vi "五参数标样核查.vi"(11 "启动参数":T1={"测量模式"=enum."水样测试", "数据标记表"="N", "输出参数"={"水温"=FALSE, "pH"=FALSE, "DO"=FALSE, "浊度"=FALSE, "电导率"=FALSE, "保存组数"=0.0}}) -> ()   [LabVIEW 2016, in "斯坦道多参数.lvlib"]
panel:
  out "枚举":T2(ring)
  out "状态":string
  out "数值":i32
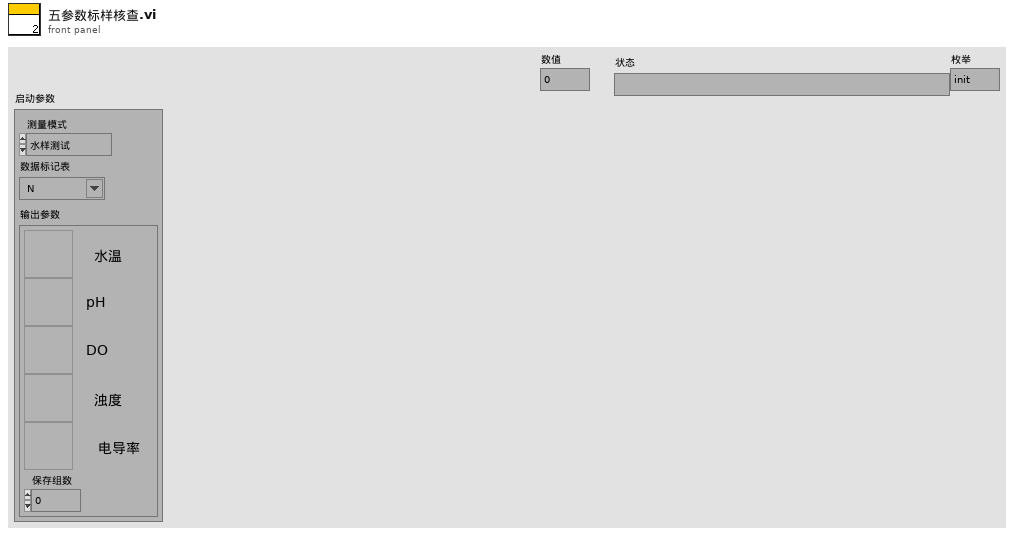
[diagram p1: front panel]
types:
  T1 = cluster{"测量模式":enum16{"待机", "水样测试", "标样核查", "零点核查", "跨度核查", "空白测试", "平行样测试", "加标回收", "空白校准", "标样校准", "初始化（清洗）"}, "数据标记表":string, "输出参数":cluster{"水温":bool, "pH":bool, "DO":bool, "浊度":bool, "电导率":bool, "保存组数":dbl}}
  T2 = enum16{"init", "开机", "启动测量", "读取测量值", "存储数据", "关闭测量", "关机", "结束"}
  T3 = cluster{"时间标识":timestamp, "设备":string, "日志信息":string, "流程参数":string}
  T4 = cluster{"系统时间":timestamp, "工作状态":u16, "测量模式":u16, "告警代码":enum16{"无告警", "缺试剂告警", "缺水样告警", "缺蒸馏水告警", "缺标液告警", "仪表漏液告警", "标定异常告警", "超量程告警", "加热异常", "低试剂预警", "超上限告警", "超下限告警", "仪表内部其他异常", "滴定异常告警", "电极异常告警", "量程切换告警", "参数设置告警", "PH电极电位异常", "电导率电极异常", "浊度光度异常", "溶解氧电极异常", "溶解氧光强异常", "温度异常告警", "PH异常告警", "溶解氧异常告警", "电导率异常告警", "浊度异常告警", "叶绿素异常告警", "藻密度异常告警", "蓝绿藻异常告警", "ORP异常告警", "氨氮异常告警", "清洁刷异常告警", "SD卡异常告警", "蓝牙异常告警", "Wifi异常告警", "流程异常告警"}, "故障代码":enum16{"无故障", "电机故障", "温度故障", "通讯故障", "滴定故障"}, "日志代码":u16, "软件版本":string}
  T5 = enum16{"待机", "水样测试", "标样核查", "零点核查", "跨度核查", "空白测试", "平行样测试", "加标回收", "空白校准", "标样校准", "初始化（清洗）"}
  T6 = cluster{"数据标记表":string, "测量模式":enum16{"待机", "水样测试", "标样核查", "零点核查", "跨度核查", "空白测试", "平行样测试", "加标回收", "空白校准", "标样校准", "初始化（清洗）"}, "database":string}
  T7 = cluster{"水温标准液标准浓度":dbl, "酸碱度标准液标准浓度":dbl, "溶解氧标准液标准浓度":dbl, "电导率标准液标准浓度":dbl, "浊度标准液标准浓度":dbl}
  T8 = cluster{"因子编码":string, "单位":string, "标样参考值":sgl, "水样数据时间":timestamp, "水样实测值":sgl, "水样数据标识":string, "K":sgl, "B":sgl, "T":sgl, "H":sgl, "水深":sgl, "探头温度":sgl}
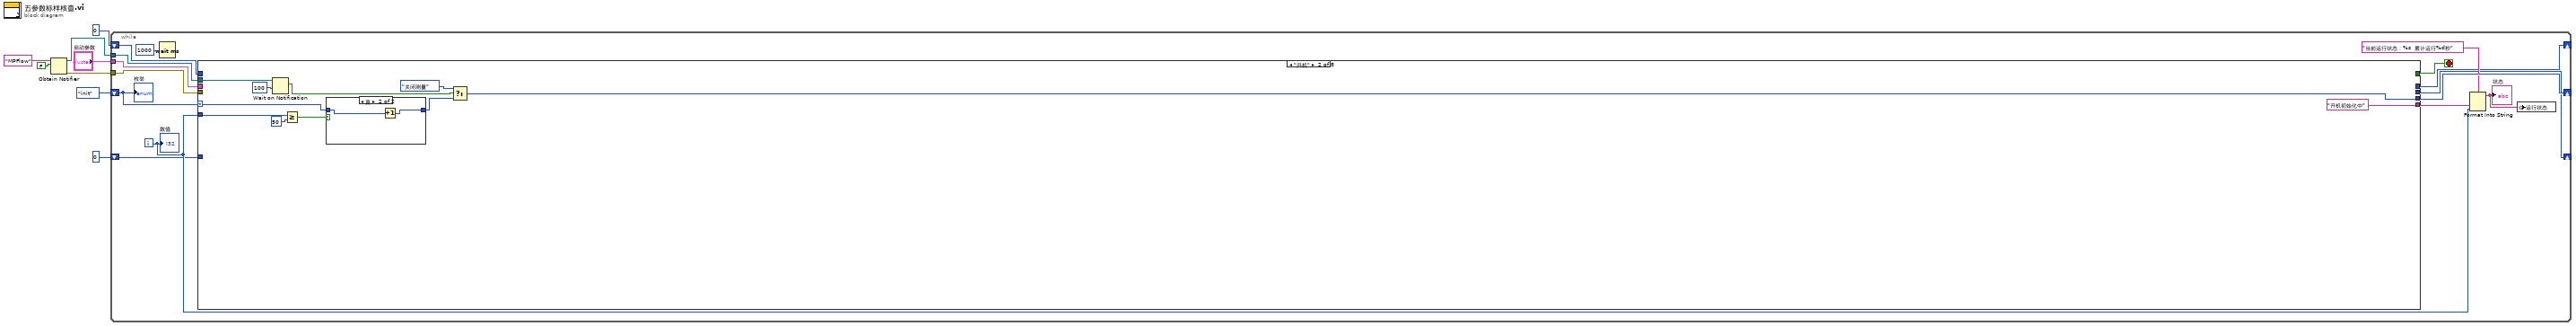
[diagram p0: block diagram]
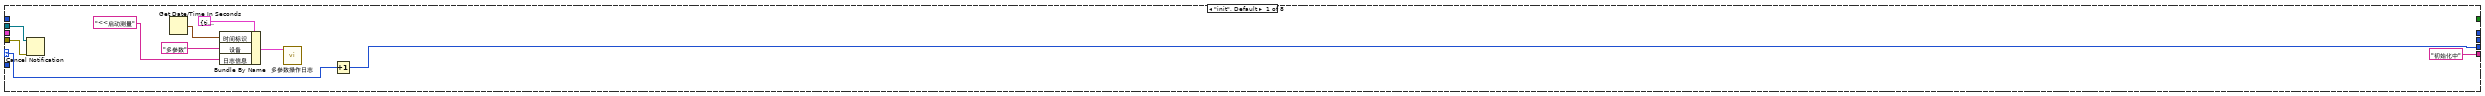
[diagram p2: hidden frame]
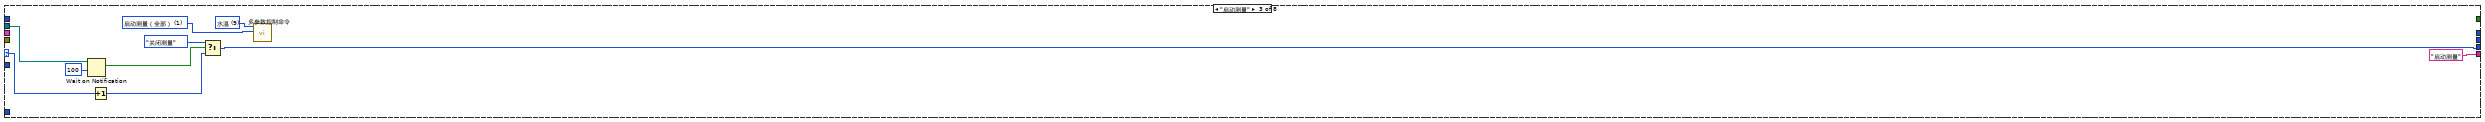
[diagram p4: hidden frame]
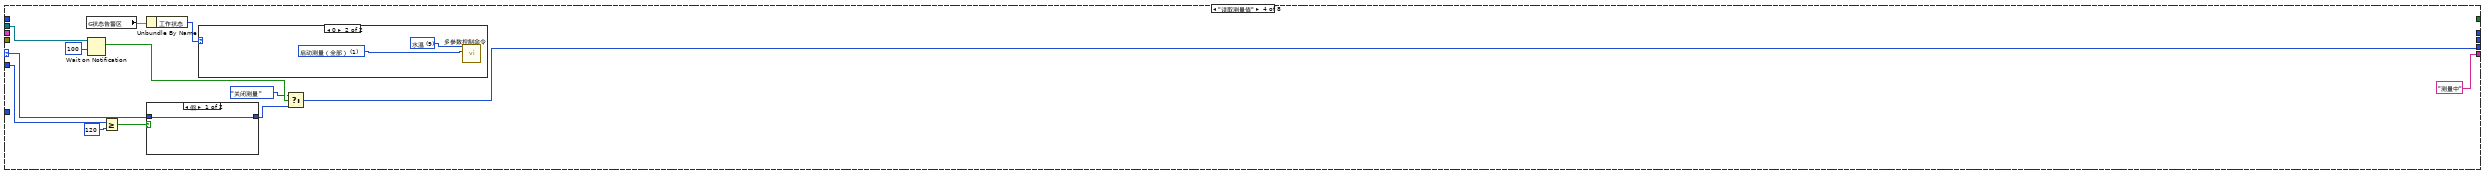
[diagram p5: hidden frame]
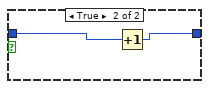
[diagram p7: hidden frame]
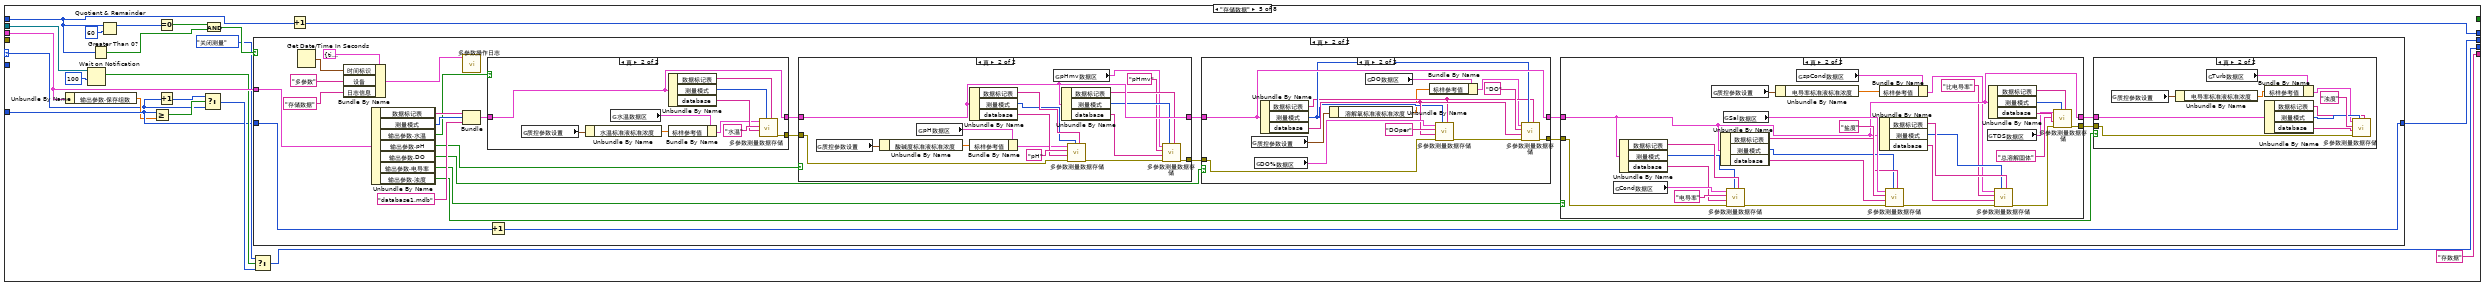
[diagram p8: hidden frame]
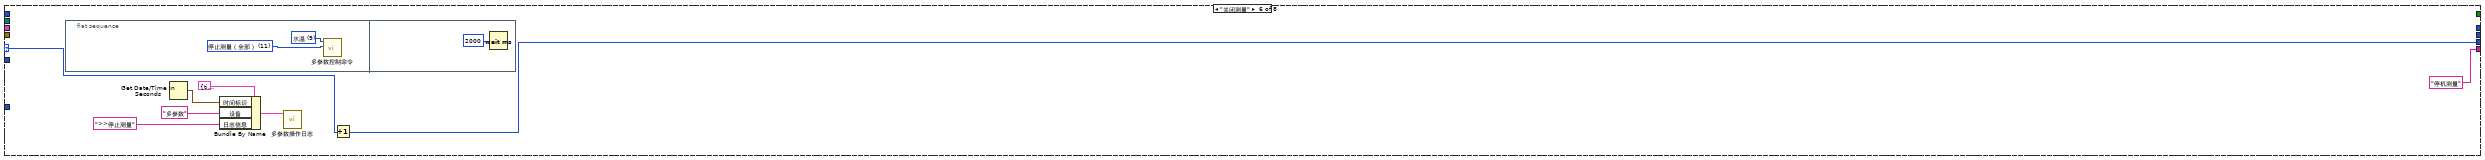
[diagram p15: hidden frame]
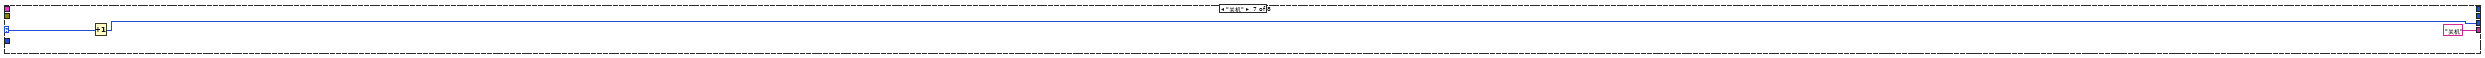
[diagram p16: hidden frame]
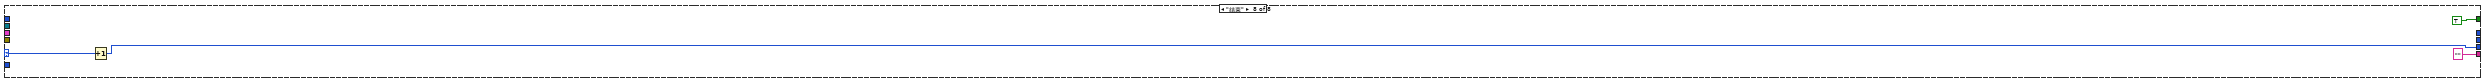
[diagram p17: hidden frame]
diagram:
  n1 = Obtain Notifier(name (unnamed)="MPFlow" ("名称（未命名）"), notification data type=FALSE) -> (notifier out=w5:refnum<notifier>, error out=w4:errorcluster)  [unwired: 2 in, 1 out]
  n2 = while {
    shift-right: [w19] -> _
    shift-left: T2."init" ("枚举") -> [w23]
    tunnel: w5 -> [w21]
    tunnel: w4 -> [w20]
    tunnel: "启动参数" -> [w13]
    shift-right: [w11] -> _
    shift-left: u32 0 ("等待时间（毫秒）") -> [w12]
    shift-right: [w9] -> _
    shift-left: u32 0 ("等待时间（毫秒）") -> [w10]
    i -> [w15]
    stop <- w22 stop-if-true
    n3 = Wait (ms)(milliseconds to wait=u32 1000 ("等待时间（毫秒）")) -> ()  [unwired: 1 out]
    n4 = case shown="\"开机\"" w23 {
      selector: w23 -> [w31 w44 w57 w70 w76 w214 w220 w223]
      tunnel: [_ _ _ _ _ _ _ TRUE] -> w22
      tunnel: w21 -> [w33 w39 w56 w67 w86 _ _ _]
      tunnel: w20 -> [w32 _ _ _ _ _ _ _]
      tunnel: [w30 w37 w53 w65 w82 w213 w219 w222] -> w19
      tunnel: w15 -> [_ w43 _ w60 _ _ _ _]
      tunnel: ["初始化中" ("状态") "开机初始化中" ("状态") "启动测量" ("状态") "测量中" ("状态") "存数据" ("状态") "停机测量" ("状态") "关机" ("状态") "" ("状态")] -> w16
      tunnel: w13 -> [_ _ _ _ w95 _ _ _]
      tunnel: w12 -> [_ _ _ _ w89 _ _ _]
      tunnel: [_ _ _ _ w90 _ _ _] -> w11
      tunnel: w10 -> [_ _ _ _ w79 _ _ _]
      tunnel: [_ _ _ _ w81 _ _ _] -> w9
      frame "init", Default {
        n5 = Cancel Notification(0:w33, 3:w32) -> ()  [unwired: 3 out]
        n6 = Get Date/Time In Seconds() -> (seconds since 1Jan1904=w27:timestamp)
        n7 = Bundle By Name(cluster=T3 {"时间标识"=timestamp(0 s since 1904-01-01), "设备"="", "日志信息"="", "流程参数"=""} ("data in"), "时间标识"=w27, "设备"="多参数", "日志信息"="<<启动测量") -> (w26:T3)
        n8 = call "多参数操作日志.vi"("data in"=w26) -> ()  [unwired: 10 in, 1 out]
        n9 = Increment(x=w31) -> (x+1=w30:T2)
      }
      frame "开机" {
        n10 = Wait on Notification(notifier=w39, timeout in ms (-1)=100 ("超时毫秒(-1)")) -> (notification=w40:bool)  [unwired: 2 in, 3 out]
        n11 = Greater Or Equal?(x=w43, y=50) -> (x >= y?=w41:bool)
        n12 = case shown="真" w41 {
          tunnel: w44 -> [w45 w47]
          tunnel: [w45 w46] -> w38
          frame False {
          }
          frame True {
            n13 = Increment(x=w47) -> (x+1=w46:T2)
          }
        }
        n14 = Select(t=T2."关闭测量" ("枚举"), s=w40, f=w38) -> (s? t:f=w37:T2)
      }
      frame "启动测量" {
        w48 = u16 1 items=["启动测量（全部）"=1, "初始化（清洗）"=10, "停止测量（全部）"=11, "校时"=13, "启动测量（单个传感器）"=19, "停止测量（单个传感器）"=20] ("控制命令")
        w49 = u16 9 items=["氨氮"=3, "水温"=9, "pH值"=10, "溶解氧"=11, "电导率"=12, "浊度"=13, "叶绿素a"=14, "藻密度"=15, "蓝绿藻"=16, "氧化还原电位"=17, "溶解氧%"=18, "盐度"=19] ("站号")
        n15 = Wait on Notification(notifier=w56, timeout in ms (-1)=100 ("超时毫秒(-1)")) -> (notification=w55:bool)  [unwired: 2 in, 3 out]
        n16 = Increment(x=w57) -> (x+1=w54:T2)
        n17 = Select(t=T2."关闭测量" ("枚举"), s=w55, f=w54) -> (s? t:f=w53:T2)
        n18 = call "多参数控制命令.vi"("控制命令"=w48, "站号"=w49) -> ()  [unwired: 9 in, 1 out]
      }
      frame "读取测量值" {
        n19 = global read "多参数全局变量.vi" "状态告警区"() -> (w59:T4)
        n20 = Wait on Notification(notifier=w67, timeout in ms (-1)=100 ("超时毫秒(-1)")) -> (notification=w68:bool)  [unwired: 2 in, 3 out]
        n21 = Greater Or Equal?(x=w60, y=120) -> (x >= y?=w69:bool)
        n22 = Unbundle By Name(w59) -> ("工作状态"=w58:u16)
        n23 = case shown="假" w69 {
          tunnel: w70 -> [w73 w75]
          tunnel: [w73 w74] -> w66
          frame False {
          }
          frame True {
            n24 = Increment(x=w75) -> (x+1=w74:T2)
          }
        }
        n25 = case shown="0" w58 {
          frame Default {
          }
          frame 0 {
            w71 = u16 1 items=["启动测量（全部）"=1, "初始化（清洗）"=10, "停止测量（全部）"=11, "校时"=13, "启动测量（单个传感器）"=19, "停止测量（单个传感器）"=20] ("控制命令")
            w72 = u16 9 items=["氨氮"=3, "水温"=9, "pH值"=10, "溶解氧"=11, "电导率"=12, "浊度"=13, "叶绿素a"=14, "藻密度"=15, "蓝绿藻"=16, "氧化还原电位"=17, "溶解氧%"=18, "盐度"=19] ("站号")
            n26 = call "多参数控制命令.vi"("控制命令"=w71, "站号"=w72) -> ()  [unwired: 9 in, 1 out]
          }
        }
        n27 = Select(t=T2."关闭测量" ("枚举"), s=w68, f=w66) -> (s? t:f=w65:T2)
      }
      frame "存储数据" {
        n28 = Unbundle By Name(w95) -> ("输出参数.保存组数"=w78:dbl)
        n29 = Wait on Notification(notifier=w86, timeout in ms (-1)=100 ("超时毫秒(-1)")) -> (notification=w85:bool)  [unwired: 2 in, 3 out]
        n30 = Greater Than 0?(x=w89) -> (x > 0?=w88:bool)
        n31 = Quotient & Remainder(x=w89, y=u32 60) -> (x-y*floor(x/y)=w93:u32)  [unwired: 1 out]
        n32 = Greater Or Equal?(x=w79, y=w78) -> (x >= y?=w80:bool)
        n33 = Equal To 0?(x=w93) -> (x = 0?=w92:bool)
        n34 = Increment(x=w76) -> (x+1=w77:T2)
        n35 = Select(t=w77, s=w80, f=w76) -> (s? t:f=w84:T2)
        n36 = Compound Arithmetic op=AND ("复合运算")(w92, w88) -> (w91:bool)
        n37 = case shown="真" w91 {
          tunnel: w95 -> [_ w122]
          tunnel: w79 -> [w97 w99]
          tunnel: [w97 w98] -> w81
          frame False {
          }
          frame True {
            n38 = Get Date/Time In Seconds() -> (seconds since 1Jan1904=w108:timestamp)
            n39 = Bundle By Name(cluster=T3 {"时间标识"=timestamp(0 s since 1904-01-01), "设备"="", "日志信息"="", "流程参数"=""} ("data in"), "时间标识"=w108, "设备"="多参数", "日志信息"="存储数据") -> (w107:T3)
            n40 = Unbundle By Name(w122) -> ("数据标记表"=w116:string, "测量模式"=w115:T5, "输出参数.水温"=w104:bool, "输出参数.pH"=w103:bool, "输出参数.DO"=w102:bool, "输出参数.电导率"=w101:bool, "输出参数.浊度"=w100:bool)
            n41 = call "多参数操作日志.vi"("data in"=w107) -> ()  [unwired: 10 in, 1 out]
            n42 = Bundle("数据标记表"=w116, "测量模式"=w115, "database"="database1.mdb") -> (w114:T6)  [unwired: 1 in]
            n43 = case shown="真" w104 {
              tunnel: [_ w205] -> w121
              tunnel: w114 -> [w196 w204]
              tunnel: [w196 w204] -> w113
              frame False {
              }
              frame True {
                n44 = global read "多参数断电保存全局变量.vi" "质控参数设置"() -> (w199:T7)
                n45 = Unbundle By Name(w199) -> ("水温标准液标准浓度"=w198:dbl)
                n46 = global read "多参数全局变量.vi" "水温数据区"() -> (w200:T8)
                n47 = Unbundle By Name(w204) -> ("数据标记表"=w203:string, "测量模式"=w202:T5, "database"=w201:string)
                n48 = Bundle By Name(cluster=w200, "标样参考值"=w198) -> (w197:T8)
                n49 = call "多参数测量数据存储.vi"("数据标记表"=w203, "测量模式"=w202, "database"=w201, "table输入"="水温", "data in"=w197) -> ("error out"=w205:errorcluster)  [unwired: 6 in]
              }
            }
            n50 = Increment(x=w99) -> (x+1=w98:u32)
            n51 = case shown="真" w103 {
              tunnel: w121 -> [_ w195]
              tunnel: [_ w185] -> w120
              tunnel: w113 -> [w178 w190]
              tunnel: [w178 w190] -> w111
              frame False {
              }
              frame True {
                n52 = global read "多参数断电保存全局变量.vi" "质控参数设置"() -> (w182:T7)
                n53 = Unbundle By Name(w182) -> ("酸碱度标准液标准浓度"=w181:dbl)
                n54 = global read "多参数全局变量.vi" "pH数据区"() -> (w180:T8)
                n55 = Unbundle By Name(w190) -> ("数据标记表"=w193:string, "测量模式"=w192:T5, "database"=w191:string)
                n56 = Bundle By Name(cluster=w180, "标样参考值"=w181) -> (w179:T8)
                n57 = global read "多参数全局变量.vi" "pHmv数据区"() -> (w184:T8)
                n58 = Unbundle By Name(w190) -> ("数据标记表"=w189:string, "测量模式"=w188:T5, "database"=w187:string)
                n59 = call "多参数测量数据存储.vi"("数据标记表"=w193, "测量模式"=w192, "error in (no error)"=w195, "database"=w191, "table输入"="pH", "data in"=w179) -> ("error out"=w186:errorcluster)  [unwired: 5 in]
                n60 = call "多参数测量数据存储.vi"("数据标记表"=w189, "测量模式"=w188, "error in (no error)"=w186, "database"=w187, "table输入"="pHmv", "data in"=w184) -> ("error out"=w185:errorcluster)  [unwired: 5 in]
              }
            }
            n61 = case shown="真" w102 {
              tunnel: w120 -> [_ w177]
              tunnel: [_ w174] -> w119
              tunnel: [w163 w171] -> w112
              tunnel: w111 -> [w163 w171]
              frame False {
              }
              frame True {
                n62 = global read "多参数断电保存全局变量.vi" "质控参数设置"() -> (w167:T7)
                n63 = global read "多参数全局变量.vi" "DO%数据区"() -> (w173:T8)
                n64 = Unbundle By Name(w171) -> ("数据标记表"=w168:string, "测量模式"=w169:T5, "database"=w170:string)
                n65 = Unbundle By Name(w167) -> ("溶解氧标准液标准浓度"=w166:dbl)
                n66 = global read "多参数全局变量.vi" "DO数据区"() -> (w165:T8)
                n67 = Bundle By Name(cluster=w165, "标样参考值"=w166) -> (w164:T8)
                n68 = call "多参数测量数据存储.vi"("数据标记表"=w168, "测量模式"=w169, "error in (no error)"=w177, "database"=w170, "table输入"="DOper", "data in"=w173) -> ("error out"=w176:errorcluster)  [unwired: 5 in]
                n69 = call "多参数测量数据存储.vi"("数据标记表"=w168, "测量模式"=w169, "error in (no error)"=w176, "database"=w170, "table输入"="DO", "data in"=w164) -> ("error out"=w174:errorcluster)  [unwired: 5 in]
              }
            }
            n70 = case shown="真" w101 {
              tunnel: w119 -> [_ w160]
              tunnel: [_ w141] -> w118
              tunnel: w112 -> [w133 w150]
              tunnel: [w133 w150] -> w110
              frame False {
              }
              frame True {
                n71 = global read "多参数全局变量.vi" "Cond数据区"() -> (w162:T8)
                n72 = Unbundle By Name(w150) -> ("数据标记表"=w155:string, "测量模式"=w154:T5, "database"=w156:string)
                n73 = global read "多参数断电保存全局变量.vi" "质控参数设置"() -> (w137:T7)
                n74 = Unbundle By Name(w150) -> ("数据标记表"=w153:string, "测量模式"=w152:T5, "database"=w151:string)
                n75 = global read "多参数全局变量.vi" "Sal数据区"() -> (w158:T8)
                n76 = call "多参数测量数据存储.vi"("数据标记表"=w155, "测量模式"=w154, "error in (no error)"=w160, "database"=w156, "table输入"="电导率", "data in"=w162) -> ("error out"=w159:errorcluster)  [unwired: 5 in]
                n77 = Unbundle By Name(w137) -> ("电导率标准液标准浓度"=w136:dbl)
                n78 = global read "多参数全局变量.vi" "spCond数据区"() -> (w135:T8)
                n79 = Bundle By Name(cluster=w135, "标样参考值"=w136) -> (w134:T8)
                n80 = Unbundle By Name(w150) -> ("数据标记表"=w149:string, "测量模式"=w148:T5, "database"=w147:string)
                n81 = call "多参数测量数据存储.vi"("数据标记表"=w153, "测量模式"=w152, "error in (no error)"=w159, "database"=w151, "table输入"="盐度", "data in"=w158) -> ("error out"=w146:errorcluster)  [unwired: 5 in]
                n82 = global read "多参数全局变量.vi" "TDS数据区"() -> (w140:T8)
                n83 = Unbundle By Name(w150) -> ("数据标记表"=w142:string, "测量模式"=w143:T5, "database"=w144:string)
                n84 = call "多参数测量数据存储.vi"("数据标记表"=w149, "测量模式"=w148, "error in (no error)"=w146, "database"=w147, "table输入"="比电导率", "data in"=w134) -> ("error out"=w145:errorcluster)  [unwired: 5 in]
                n85 = call "多参数测量数据存储.vi"("数据标记表"=w142, "测量模式"=w143, "error in (no error)"=w145, "database"=w144, "table输入"="总溶解固体", "data in"=w140) -> ("error out"=w141:errorcluster)  [unwired: 5 in]
              }
            }
            n86 = case shown="真" w100 {
              tunnel: w118 -> [_ w132]
              tunnel: w110 -> [_ w130]
              frame False {
              }
              frame True {
                n87 = global read "多参数断电保存全局变量.vi" "质控参数设置"() -> (w126:T7)
                n88 = Unbundle By Name(w126) -> ("电导率标准液标准浓度"=w125:dbl)
                n89 = global read "多参数全局变量.vi" "Turb数据区"() -> (w124:T8)
                n90 = Bundle By Name(cluster=w124, "标样参考值"=w125) -> (w123:T8)
                n91 = Unbundle By Name(w130) -> ("数据标记表"=w127:string, "测量模式"=w128:T5, "database"=w129:string)
                n92 = call "多参数测量数据存储.vi"("数据标记表"=w127, "测量模式"=w128, "error in (no error)"=w132, "database"=w129, "table输入"="浊度", "data in"=w123) -> ()  [unwired: 5 in, 1 out]
              }
            }
          }
        }
        n93 = Select(t=T2."关闭测量", s=w85, f=w84) -> (s? t:f=w82:T2)
        n94 = Increment(x=w89) -> (x+1=w90:u32)
      }
      frame "关闭测量" {
        n95 = flat-sequence {
          frame #0 {
            w215 = u16 11 items=["启动测量（全部）"=1, "初始化（清洗）"=10, "停止测量（全部）"=11, "校时"=13, "启动测量（单个传感器）"=19, "停止测量（单个传感器）"=20] ("控制命令")
            w216 = u16 9 items=["氨氮"=3, "水温"=9, "pH值"=10, "溶解氧"=11, "电导率"=12, "浊度"=13, "叶绿素a"=14, "藻密度"=15, "蓝绿藻"=16, "氧化还原电位"=17, "溶解氧%"=18, "盐度"=19] ("站号")
            n96 = call "多参数控制命令.vi"("控制命令"=w215, "站号"=w216) -> ()  [unwired: 9 in, 1 out]
          }
          frame #1 {
            n97 = Wait (ms)(milliseconds to wait=u32 2000 ("等待时间（毫秒）")) -> ()  [unwired: 1 out]
          }
        }
        n98 = Get Date/Time In Seconds() -> (seconds since 1Jan1904=w210:timestamp)
        n99 = Bundle By Name(cluster=T3 {"时间标识"=timestamp(0 s since 1904-01-01), "设备"="", "日志信息"="", "流程参数"=""} ("data in"), "时间标识"=w210, "设备"="多参数", "日志信息"=">>停止测量") -> (w209:T3)
        n100 = call "多参数操作日志.vi"("data in"=w209) -> ()  [unwired: 10 in, 1 out]
        n101 = Increment(x=w214) -> (x+1=w213:T2)
      }
      frame "关机" {
        n102 = Increment(x=w220) -> (x+1=w219:T2)
      }
      frame "结束" {
        n103 = Increment(x=w223) -> (x+1=w222:T2)
      }
    }
    n104 = Format Into String(format string="当前运行状态：%s  累计运行%d秒" ("格式字符串"), w16, w15) -> (resulting string=w14:string)  [unwired: 2 in, 1 out]
    "状态" <- w14
    n105 = global write "多参数全局变量.vi" "运行状态"(w14) -> ()
    "数值" <- w15
    "枚举" <- w23
  }
